vi "切换增益.vi"(8 "error in":errorcluster, 10 "增益":u32) -> (0 "error out":errorcluster, 2 "return":i32)   [LabVIEW 2016]
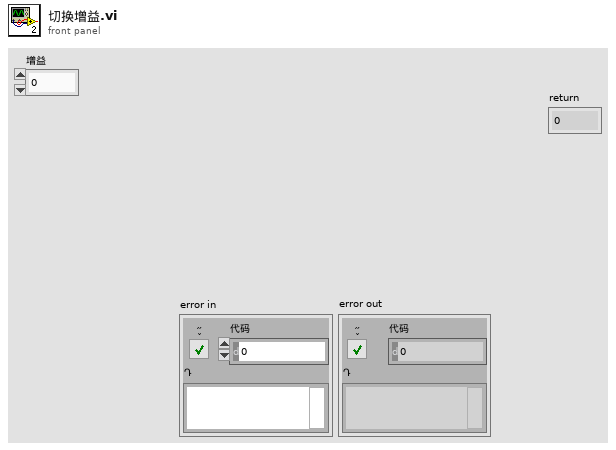
[diagram p1: front panel]
types:
  T1 = cluster{"byCmdType":u8, "bySubCmd":u8, "byParam_h":u8, "byParam_l":u8, "byAddr1_hh":u8, "byAddr1_h":u8, "byAddr1_l":u8, "byAddr1_ll":u8, "byAddr2_hh":u8, "byAddr2_h":u8, "byAddr2_l":u8, "byAddr2_ll":u8, "byLen_hh":u8, "byLen_h":u8, "byLen_l":u8, "byLen_ll":u8}
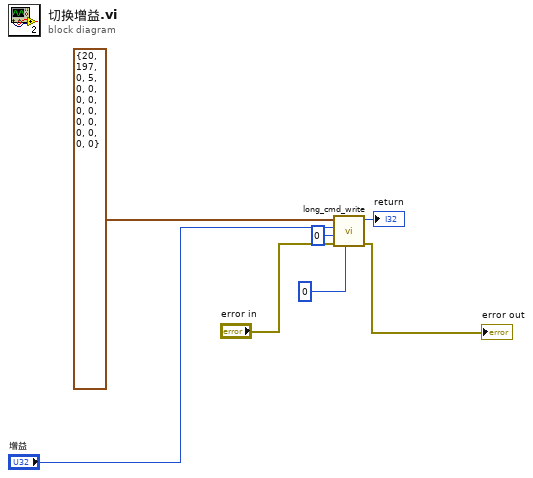
[diagram p0: block diagram]
diagram:
  n1 = call "long_cmd_write.vi"("dwLen"=u32 0, "error in"="error in", "dwAddr2"=u32 0, "dwAddr1"="增益", "vd_cmd_long_header_t"=T1 {"byCmdType"=20, "bySubCmd"=197, "byParam_h"=0, "byParam_l"=5, "byAddr1_hh"=0, "byAddr1_h"=0, "byAddr1_l"=0, "byAddr1_ll"=0, "byAddr2_hh"=0, "byAddr2_h"=0, "byAddr2_l"=0, "byAddr2_ll"=0, "byLen_hh"=0, "byLen_h"=0, "byLen_l"=0, "byLen_ll"=0}) -> ("error out"=→"error out":errorcluster, "return"=→"return":i32)  [unwired: 5 in]
